vi "Dynamic call-Larger image window.vi"(8 "error in (no error)":errorcluster, 10 "Image name":string, 11 "Open maximised":bool) -> (0 "error out":errorcluster)   [LabVIEW 2013]
uses:
  Visualisation/Timelapse Viewer/Globals/gl_Time series viewer globals.vi
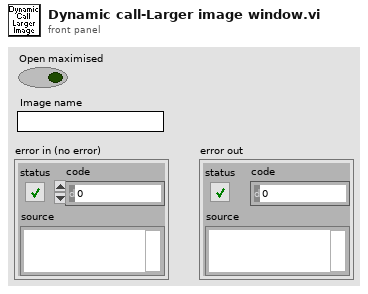
[diagram p1: front panel]
types:
  T1 = enum16{"None", "Release queue", "Obtain queue", "Enqueue", "Get status", "Set status"}
  T2 = typedef "Larger windows queues interface cluster.ctl" = cluster{"error out 1":errorcluster, "Window 1 is open":bool, "error out 2":errorcluster, "Window 2 is open":bool, "error out 3":errorcluster, "Window 3 is open":bool, "error out 4":errorcluster, "Window 4 is open":bool, "Larger image window queue 1":T3, "Larger image window queue 2":T3, "Larger image window queue 3":T3, "Larger image window queue 4":T3}
  T3 = typedef "Larger window queue ref.ctl" = refnum<queue>
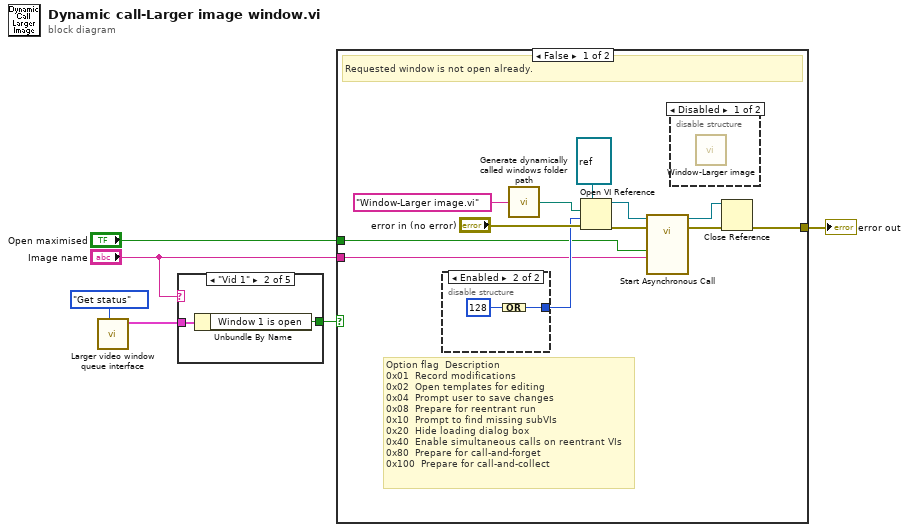
[diagram p0: block diagram]
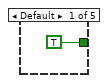
[diagram p2: hidden frame]
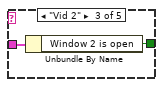
[diagram p3: hidden frame]
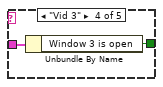
[diagram p4: hidden frame]
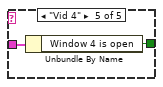
[diagram p5: hidden frame]
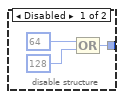
[diagram p6: hidden frame]
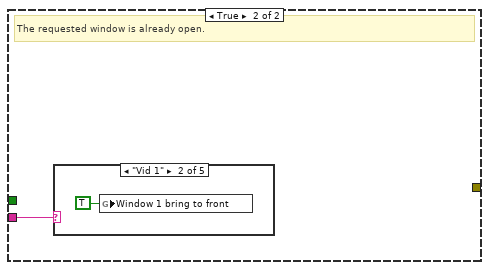
[diagram p8: hidden frame]
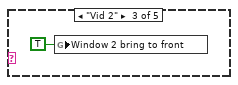
[diagram p10: hidden frame]
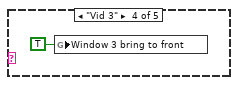
[diagram p11: hidden frame]
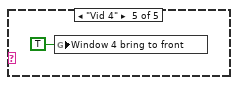
[diagram p12: hidden frame]
diagram:
  n1 = call "Larger video window queue interface.vi"("Function"=T1."Get status") -> ("Output cluster"=w4:T2)  [unwired: 10 in]
  n2 = case shown="\"Vid 1\"" "Image name" {
    tunnel: w4 -> [_ w9 w11 w13 w15]
    tunnel: [TRUE ("Window 4 is open") w8 w10 w12 w14] -> w3
    frame Default {
    }
    frame "Vid 1" {
      n3 = Unbundle By Name(w9) -> ("Window 1 is open"=w8:bool)
    }
    frame "Vid 2" {
      n4 = Unbundle By Name(w11) -> ("Window 2 is open"=w10:bool)
    }
    frame "Vid 3" {
      n5 = Unbundle By Name(w13) -> ("Window 3 is open"=w12:bool)
    }
    frame "Vid 4" {
      n6 = Unbundle By Name(w15) -> ("Window 4 is open"=w14:bool)
    }
  }
  n7 = case shown="False" w3 {
    tunnel: [w26 _] -> w6
    tunnel: "Image name" -> [w17 w33]
    tunnel: "Open maximised" -> [w16 _]
    frame False {
      # "Option flag \tDescription\n0x01 \tRecord modifications\n0x02 \tOpen templates for editing\n0x04 \tPrompt user to save changes\n0x08 \tPrepare for reentrant run\n0x10 \tPrompt to find missing subVIs\n0x20 \tHide loading dialog box\n0x40 \tEnable simultaneous calls on reentrant VIs\n0x80 \tPrepare for call-and-forget\n0x100 \tPrepare for call-and-collect"
      # "Requested window is not open already."
      n8 = disable-structure shown="Enabled" {
        disable-tunnel: [w30 w32] -> w21
        frame Disabled {
          n9 = Compound Arithmetic op=OR(64, 128) -> (w30:i32)
        }
        frame Enabled {
          n10 = Compound Arithmetic op=OR(128) -> (w32:i32)
        }
      }
      n11 = call "Generate dynamically called windows folder path.vi"("name of dynamically called VI"="Window-Larger image.vi" ("Error Source")) -> ("Dynamically called VI path"=w25:path)
      n12 = Open VI Reference(type specifier VI Refnum (for type only)=refnum<vi> refnum, vi path=w25, options=w21, error in (no error)="error in (no error)") -> (vi reference=w22:refnum<vi>, error out=w23:errorcluster)  [unwired: 2 in]
      n13 = call-by-ref "Start Asynchronous Call"(reference=w22, error in=w23, "Image name"=w17, "Open maximised"=w16) -> (reference out=w18:refnum<vi>, error out=w19:errorcluster)  [unwired: 10 in]
      n14 = disable-structure shown="Disabled" {
        frame Disabled {
          n15 = call "Window-Larger image.vi"() -> ()  [unwired: 12 in]
        }
        frame Enabled {
        }
      }
      n16 = Close Reference(reference=w18, error in (no error)=w19) -> (error out=w26:errorcluster)
    }
    frame True {
      # "The requested window is already open."
      n17 = case shown="\"Vid 1\"" w33 {
        frame Default {
        }
        frame "Vid 1" {
          n18 = global write "gl_Time series viewer globals.vi" "Window 1 bring to front"(TRUE ("Window 1 bring to front")) -> ()
        }
        frame "Vid 2" {
          n19 = global write "gl_Time series viewer globals.vi" "Window 2 bring to front"(TRUE ("Window 2 bring to front")) -> ()
        }
        frame "Vid 3" {
          n20 = global write "gl_Time series viewer globals.vi" "Window 3 bring to front"(TRUE ("Window 3 bring to front")) -> ()
        }
        frame "Vid 4" {
          n21 = global write "gl_Time series viewer globals.vi" "Window 4 bring to front"(TRUE ("Window 4 bring to front")) -> ()
        }
      }
    }
  }
  "error out" <- w6
